vi "Convert HW file path to paramID path.vi"(8 "error in (no error)":errorcluster, 11 "Hw File In":path) -> (0 "error out":errorcluster, 2 "Param Id File out":path, 3 "Hw File Out":path)   [LabVIEW 2020, in "Ballard 1553 System Explorer.lvlib"]
uses:
  Ballard 1553 System Explorer.lvlib
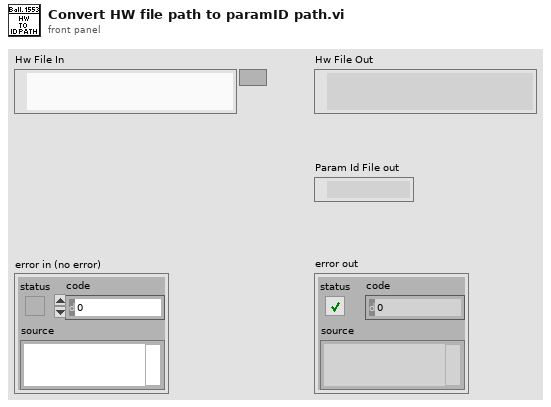
[diagram p1: front panel]
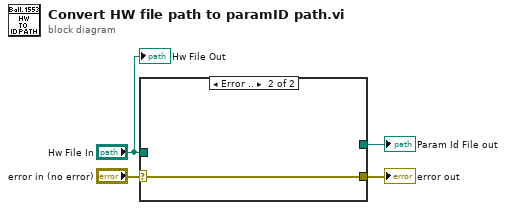
[diagram p0: block diagram]
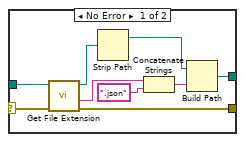
[diagram p2: hidden frame]
diagram:
  n1 = case shown="Error .." "error in (no error)" {
    selector: "error in (no error)" -> [w8 w14]
    tunnel: "Hw File In" -> [w7 _]
    tunnel: [w6 w14] -> w2
    tunnel: [w5 _] -> w1
    frame No Error {
      n2 = call <vilib>:"Get File Extension.vi"("error in (no error)"=w8, "file"=w7) -> ("error out"=w6:errorcluster, "filename without extension"=w11:string, "dup file"=w13:path)  [unwired: 5 in, 2 out]
      n3 = Strip Path(path=w13) -> (stripped path=w12:path)  [unwired: 1 out]
      n4 = Concatenate Strings(w11, ".json" ("string")) -> (w9:string)
      n5 = Build Path(base path=w12, name or relative path=w9) -> (appended path=w5:path)
    }
    frame Error {
    }
  }
  "error out" <- w2
  "Param Id File out" <- w1
  "Hw File Out" <- "Hw File In"
